vi "N 2DGaussianRotationModel.vi"(3 "output control":T1, 4 "data":T2, 5 "X":dbl[](array[numeric]), 6 "a":dbl[](array[numeric])) -> (0 "error out":errorcluster, 1 "f'(X,a)":dbl[][](array[numeric]), 2 "f(X,a)":dbl[](array[numeric]))   [LabVIEW 2011]
doc: "This template is the starting point for creating a model function to be passed to the Nonlinear Curve Fit.vi."
uses:
  <vilib>/gmath/NumericalOptimization/objective function data.ctl
  <vilib>/gmath/NumericalOptimization/LM_output select.ctl
  <vilib>/gmath/NI_Gmath.lvlib
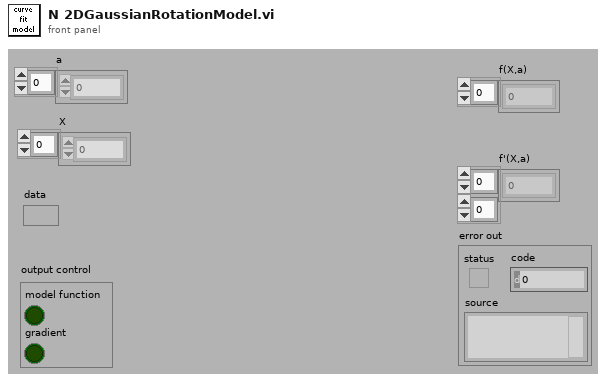
[diagram p1: front panel]
types:
  T1 = typedef "NI_Gmath.lvlib/LM_output select.ctl" = cluster{"model function":bool, "gradient":bool}
  T2 = typedef "NI_Gmath.lvlib/objective function data.ctl" = variant
  T3 = cluster{"Width":i32, "Height":i32, "N Gaussians":i32}
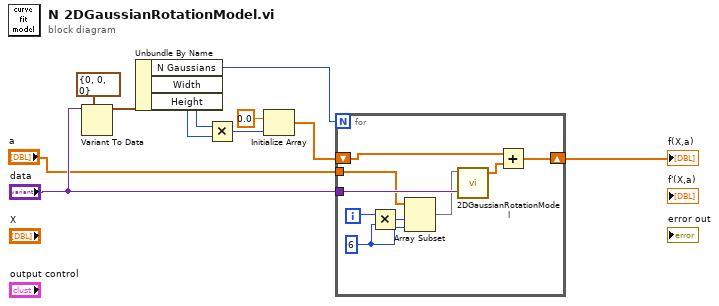
[diagram p0: block diagram]
diagram:
  n1 = Variant To Data(type=T3 {"Width"=0, "Height"=0, "N Gaussians"=0} ("Plot Area:Size"), Variant="data") -> (data=w10:T3)  [unwired: 1 in, 1 out]
  n2 = Unbundle By Name(w10) -> ("N Gaussians"=w1:i32, "Width"=w5:i32, "Height"=w4:i32)
  n3 = Multiply(x=w5, y=w4) -> (x*y=w3:i32)
  n4 = Initialize Array(0.0 ("element"), w3) -> (w6:dbl[])
  n5 = for {
    N: w1 -> [_]
    tunnel: "data" -> [w20]
    shift-right: [w18] -> w11
    shift-left: w6 -> [w17]
    tunnel: "a" -> [w16]
    i -> [w14]
    w13 = 6 ("x")
    n6 = Multiply(x=w14, y=w13) -> (x*y=w15:i32)
    n7 = Array Subset(array=w16, index=w15, length=w13) -> (w12:dbl[])
    n8 = call "2DGaussianRotationModel.vi"("data"=w20, "a"=w12) -> ("f(X,a)"=w19:dbl[])  [unwired: 2 in, 2 out]
    n9 = Add(x=w17, y=w19) -> (x+y=w18:dbl[])
  }
  "f(X,a)" <- w11
